vi "From Pythonic - Boolean Array.vi"(4 "Pythonic Value":string) -> (1 "Boolean Array":bool[](array[boolean]))   [LabVIEW 2012, in "OPI.lvclass"]
doc: "Convert pythonic values into LabVIEW data. This method can be helpfull to convert elements of tuples or dictionaries.\n\nReturn a 1D array of boolean."
uses:
  OPI.lvclass
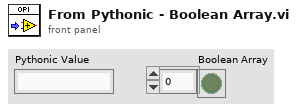
[diagram p1: front panel]
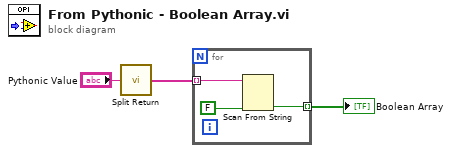
[diagram p0: block diagram]
diagram:
  n1 = call "Split Return.vi"("Return Value"="Pythonic Value") -> ("Split String"=w3:string[])
  n2 = for {
    tunnel: [w5] -> w2 mode=indexing
    tunnel: w3 -> [w4] mode=indexing
    n3 = Scan From String(input string=w4, default 1=FALSE) -> (output 1=w5:bool)  [unwired: 3 in, 3 out]
  }
  "Boolean Array" <- w2
